vi "AnyBuilderBeginNestedMessage.vi"(8 "error in":errorcluster, 10 "protobufId":i32, 11 "gRPCid in":T1) -> (0 "error out":errorcluster, 2 "Nested ID":T1, 3 "gRPCid out":T1)   [LabVIEW 2019, in "grpc-lvsupport.lvlib"]
uses:
  grpc-lvsupport.lvlib
  Shared/grpcId.ctl
  <vilib>/Utility/error.llb/Error Cluster From Error Code.vi
  <resource>/labview_grpc_server.dll
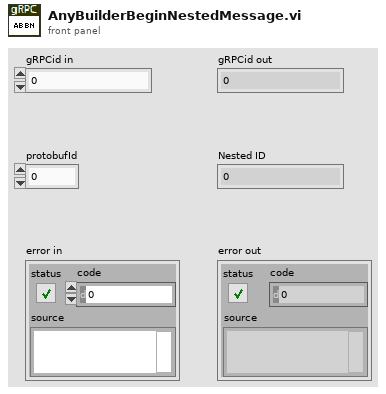
[diagram p1: front panel]
types:
  T1 = typedef "grpc-lvsupport.lvlib/grpcId.ctl" = u64
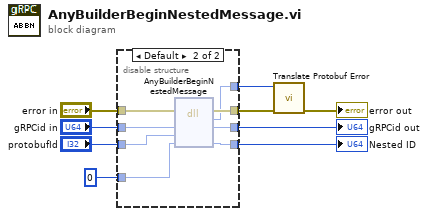
[diagram p0: block diagram]
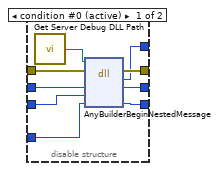
[diagram p2: hidden frame]
diagram:
  n1 = disable-structure shown="Default" {
    disable-tunnel: "error in" -> [w18 w26]
    disable-tunnel: [w17 w25] -> w8
    disable-tunnel: "protobufId" -> [w16 w24]
    disable-tunnel: "gRPCid in" -> [w15 w23]
    disable-tunnel: [w14 w22] -> w5
    disable-tunnel: [w12 w21] -> w4
    disable-tunnel: u64 0 ("nestedId") -> [w11 w20]
    disable-tunnel: [w10 w19] -> w1
    frame condition #0 (active) {
      n2 = call "Get Server Debug DLL Path.vi"() -> ("Server Debug DLL Path"=w13:path)
      n3 = dll-call lib="?" fn="AnyBuilderBeginNestedMessage"(path in=w13, error in=w18, "builderId"=w15, "protobufId"=w16, "nestedId"=w11) -> (error out=w17:errorcluster, "return type"=w10:i32, "builderId"=w14:u64, "nestedId"=w12:u64)  [unwired: 2 in, 1 out]
    }
    frame condition #1 {
      n4 = dll-call lib="C:/Program Files (x86)/National Instruments/LabVIEW 2024/resource/labview_grpc_server.*" fn="AnyBuilderBeginNestedMessage"(error in=w26, "builderId"=w23, "protobufId"=w24, "nestedId"=w20) -> (error out=w25:errorcluster, "return type"=w19:i32, "builderId"=w22:u64, "nestedId"=w21:u64)  [unwired: 3 in, 1 out]
    }
  }
  "gRPCid out" <- w5
  "Nested ID" <- w4
  n5 = call "Translate Protobuf Error.vi"("error in"=w8, "Error Code"=w1) -> ("error out"=→"error out":errorcluster)  [unwired: 9 in]
